vi "Change_Aperence_of_the_Menu_Items.vi"(5 "VI Ref":refnum<vi>, 6 "Button_Color_Off":u32=2344, 7 "Button_Color_On":u32=5654, 8 "error in":errorcluster, 9 "Panel_Color":u32=2344, 10 "Button_Label_Color":u32=2344, 11 "Menu":refnum<vi>) -> (0 "error out":errorcluster)   [LabVIEW 2019]
doc: "Change the Apperence of the Menu\nThis will change\nText Color\nCluster BG Color\nButton ON/OFF Color\n\nAll Rights Reserved © 2017 SyncSols"
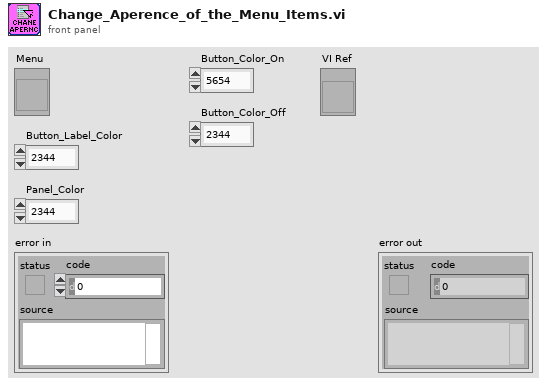
[diagram p1: front panel]
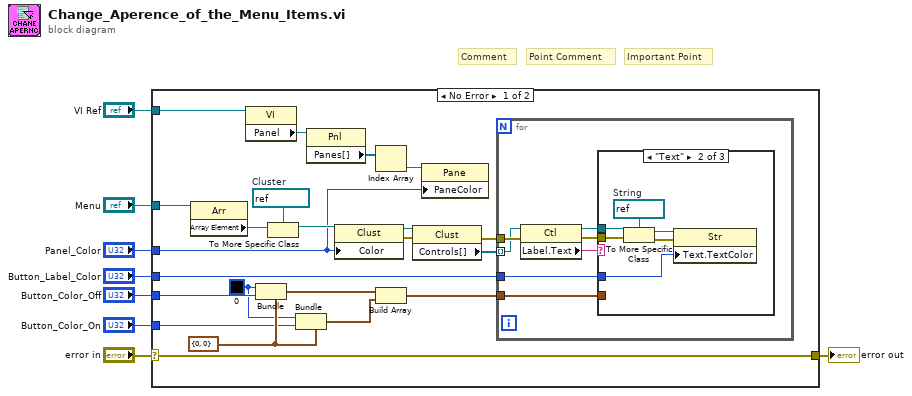
[diagram p0: block diagram]
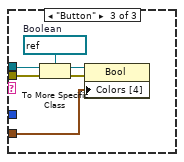
[diagram p3: hidden frame]
diagram:
  # "Important Point"
  # "Point Comment"
  # "Comment"
  n1 = case shown="No Error" "error in" {
    selector: "error in" -> [w30 w50]
    tunnel: [w30 w50] -> w8
    tunnel: "Menu" -> [w29 _]
    tunnel: "Panel_Color" -> [w10 _]
    tunnel: "Button_Label_Color" -> [w21 _]
    tunnel: "Button_Color_Off" -> [w20 _]
    tunnel: "Button_Color_On" -> [w18 _]
    tunnel: "VI Ref" -> [w9 _]
    frame No Error {
      w17 = u32 0
      w19 = cluster{u32, u32} {0, 0}
      w27 = refnum<vi> refnum  # Cluster
      n2 = property class="Arr"(reference=w29) -> ("Array Element"=w28:refnum<vi>)  [unwired: 1 in, 2 out]
      n3 = property class="VI"(reference=w9) -> ("Panel"=w13:refnum<vi>)  [unwired: 1 in, 2 out]
      n4 = Bundle(cluster=w19, w17, w20) -> (w16:cluster{u32, u32})
      n5 = To More Specific Class(target class=w27, reference=w28) -> (specific class reference=w26:refnum<vi>)  [unwired: 1 in, 1 out]
      n6 = Bundle(cluster=w19, w17, w18) -> (w15:cluster{u32, u32})
      n7 = property class="Pnl"(reference=w13) -> ("Panes[]"=w12:refnum<vi>[])  [unwired: 1 in, 2 out]
      n8 = property class="Clust"(reference=w26, "Color"=w10) -> (reference out=w25:refnum<vi>, error out=w24:errorcluster)  [unwired: 1 in]
      n9 = Index Array(array=w12) -> (element=w11:refnum<vi>)  [unwired: 1 in]
      n10 = Build Array(w16, w15) -> (w14:cluster{u32, u32}[])
      n11 = property class="Clust"(reference=w25, error in=w24) -> (error out=w22:errorcluster, "Controls[]"=w23:refnum<vi>[])  [unwired: 1 out]
      n12 = property class="Pane"(reference=w11, "PaneColor"=w10) -> ()  [unwired: 1 in, 2 out]
      n13 = for {
        tunnel: w23 -> [w36] mode=indexing
        tunnel: w22 -> [w37]
        tunnel: w21 -> [w32]
        tunnel: w14 -> [w31]
        n14 = property class="Ctl"(reference=w36, error in=w37) -> (reference out=w33:refnum<vi>, error out=w34:errorcluster, "Label.Text"=w35:string)
        n15 = case shown="\"Text\"" w35 {
          tunnel: w34 -> [_ w43 w48]
          tunnel: w33 -> [_ w42 w47]
          tunnel: w32 -> [_ w39 _]
          tunnel: w31 -> [_ _ w44]
          frame "False", Default {
          }
          frame "Text" {
            w41 = refnum<vi> refnum  # String
            n16 = To More Specific Class(target class=w41, reference=w42, error in=w43) -> (specific class reference=w40:refnum<vi>, error out=w38:errorcluster)
            n17 = property class="Str"(reference=w40, error in=w38, "Text.TextColor"=w39) -> ()  [unwired: 2 out]
          }
          frame "Button" {
            w49 = refnum<vi> refnum  # Boolean
            n18 = To More Specific Class(target class=w49, reference=w47, error in=w48) -> (specific class reference=w46:refnum<vi>, error out=w45:errorcluster)
            n19 = property class="Bool"(reference=w46, error in=w45, "Colors [4]"=w44) -> ()  [unwired: 2 out]
          }
        }
      }
    }
    frame Error {
    }
  }
  "error out" <- w8
